vi "ROI entry-Actions on all ROI cleared.vi"(11 "No ROIs (T)":bool=TRUE) -> ()   [LabVIEW 2013]
uses:
  ROI Entry screen/Typedefs/ROI input mode.ctl
  ROI Entry screen/Globals/gl_ROI Entry UI globals.vi
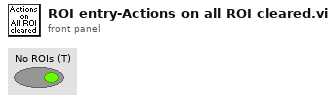
[diagram p1: front panel]
types:
  T1 = enum8{"Enabled", "Disabled", "Disabled and Grayed Out"}
  T2 = typedef "ROI input mode.ctl" = enum16{"Unspecified", "Point-Line-Plane", "Volume"}
  T3 = typedef "IMAQ Image.ctl" = refnum<image>
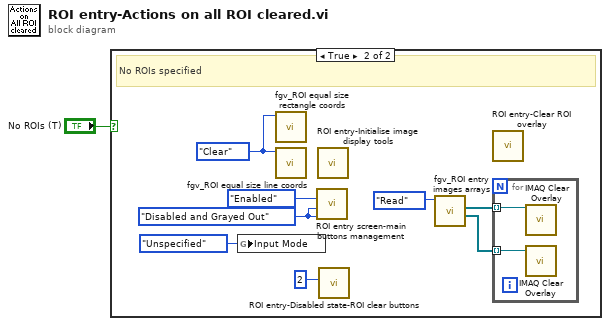
[diagram p0: block diagram]
diagram:
  n1 = case shown="True" "No ROIs (T)" {
    frame False {
      # "Some ROI still exist"
    }
    frame True {
      w2 = enum16{"Intialize", "Write", "Read", "Clear"}."Clear" ("Function")
      w9 = T1."Disabled and Grayed Out" ("Disabled")
      # "No ROIs specified"
      n2 = global write "gl_ROI Entry UI globals.vi" "Input Mode"(ROI_input_mode."Unspecified" ("Input Mode")) -> ()
      n3 = call "fgv_ROI equal size rectangle coords.vi"("Function"=w2) -> ()  [unwired: 9 in, 2 out]
      n4 = call "fgv_ROI equal size line coords.vi"("Function"=w2) -> ()  [unwired: 9 in, 2 out]
      n5 = call "ROI entry screen-main buttons management.vi"("Imaging button disabled?"=w9, "Acquisition button disabled?"=w9, "Done button disabled?"=T1."Enabled") -> ()  [unwired: 9 in]
      n6 = call "ROI entry-Initialise image display tools.vi"() -> ()  [unwired: 11 in, 1 out]
      n7 = call "ROI entry-Disabled state-ROI clear buttons.vi"("State"=2) -> ()  [unwired: 10 in, 1 out]
      n8 = call "fgv_ROI entry images arrays.vi"("Function"=enum16{"Intialize", "Write", "Read", "Clear"}."Read") -> ("GreenImageArray"=w5:T3[], "RedImageArray"=w4:T3[])  [unwired: 8 in, 1 out]
      n9 = call "ROI entry-Clear ROI overlay.vi"() -> ()  [unwired: 10 in, 2 out]
      n10 = for {
        tunnel: w4 -> [w11] mode=indexing
        tunnel: w5 -> [w10] mode=indexing
        n11 = call "IMAQ Clear Overlay"("Image"=w11) -> ()  [unwired: 9 in, 2 out]
        n12 = call "IMAQ Clear Overlay"("Image"=w10) -> ()  [unwired: 9 in, 2 out]
      }
    }
  }
